vi "PR_Replace_data.vi"(7 "Boolean":bool, 8 "error in (no error)":errorcluster, 9 "Barcode_B":string, 10 "Barcode_A":string, 11 "DBlink":string="Driver={ODBC Driver 17 for SQL Server};Server=localhost\\SQLEXPRESS;Database=ZDX201;UID=labview;PWD=Dsa@54137926") -> (0 "error out":errorcluster, 1 "data":cluster{string}[](array[cluster]))   [LabVIEW 2019]
uses:
  <vilib>/addons/database/Connection.llb/DB Tools Open Connec (String).vi
  <vilib>/addons/database/Connection.llb/Conn Execute.vi
  <vilib>/addons/database/Recordset.llb/Rec Fetch Recordset Data (R).vi
  <vilib>/addons/database/Recordset.llb/Rec Destroy - Connection.vi
  <vilib>/addons/database/_DB Variant To Data/Database Variant To Data.xnode
  <vilib>/addons/database/NI_Database_API.lvlib
panel:
  out "Command 1":string="SELECT TOP (1) [id]      \n FROM [ZDX201].[dbo].[glue_data]\n where glue_workspace_id=4\nand evaluation_1 is null\norder by id desc "
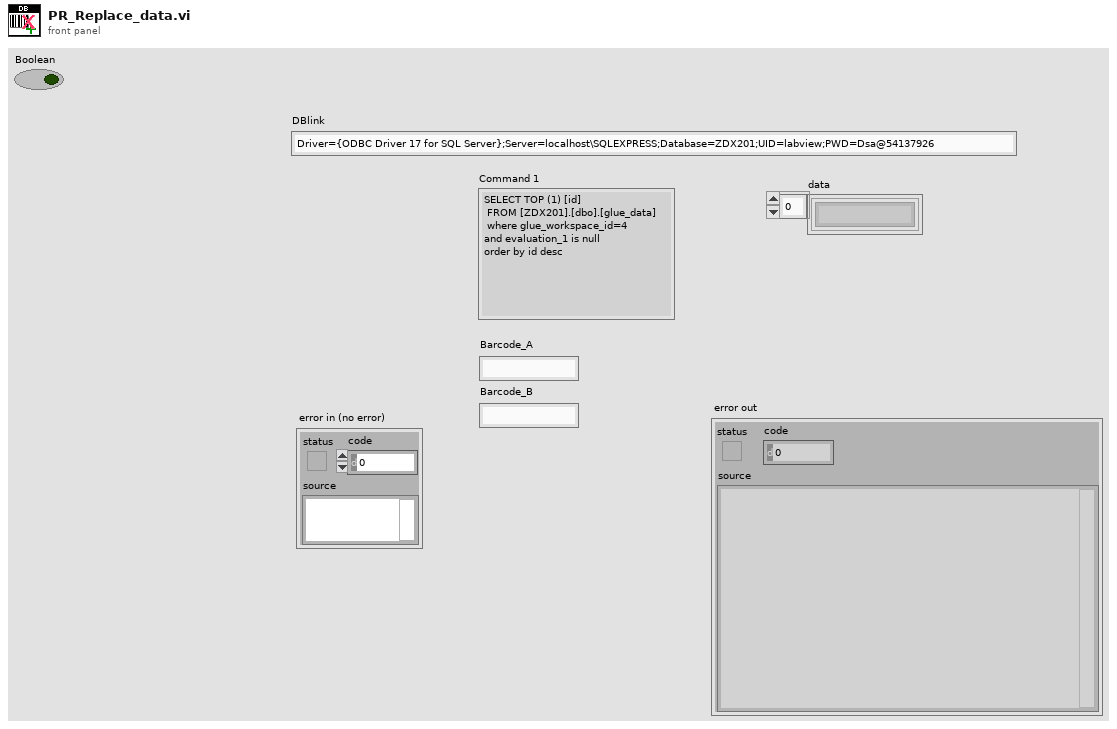
[diagram p1: front panel]
types:
  T1 = typedef "NI_Database_API.lvlib/Conn ObjectReference.ctl" = refnum<k1>
  T2 = typedef "NI_Database_API.lvlib/Rec ObjectReference.ctl" = refnum<k1>
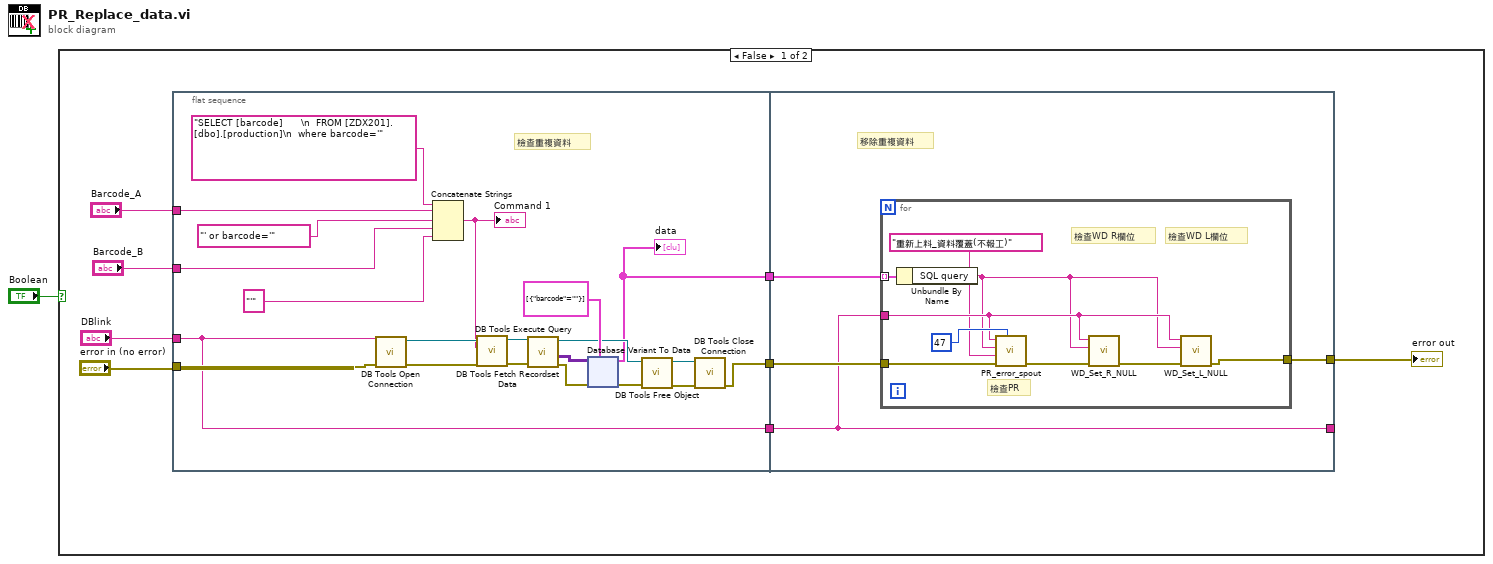
[diagram p0: block diagram]
diagram:
  n1 = case shown="False" "Boolean" {
    frame False {
      n2 = flat-sequence {
        tunnel: "DBlink" -> [w18]
        tunnel: "error in (no error)" -> [w30]
        tunnel: [w19] -> w7
        tunnel: [w18] -> w6
        tunnel: [w12] -> w5
        tunnel: "Barcode_A" -> [w11]
        tunnel: "Barcode_B" -> [w10]
        tunnel: [w74] -> _
        tunnel: w7 -> [w75]
        tunnel: w6 -> [w74]
        tunnel: w5 -> [w73]
        tunnel: [w72] -> w2
        frame #0 {
          # "檢查重複資料"
          n3 = call-poly <vilib>:"DB Tools Open Connection.vi"("error in (no error)"=w30, "connection information"=w18) -> ("error out"=w29:errorcluster, "connection reference"=w28:T1)  [unwired: 6 in]
          n4 = Concatenate Strings("SELECT [barcode]      \n  FROM [ZDX201].[dbo].[production]\n  where barcode='" ("SQL query"), w11, "' or barcode='" ("SQL query"), w10, "'" ("SQL query")) -> (w13:string)
          "Command 1" <- w13
          n5 = call-poly <vilib>:"DB Tools Execute Query.vi"("error in (no error)"=w29, "SQL query"=w13, "connection reference"=w28) -> ("error out"=w27:errorcluster, "recordset reference"=w26:T2)  [unwired: 5 in]
          n6 = call-poly <vilib>:"DB Tools Fetch Recordset Data.vi"("error in (no error)"=w27, "recordset reference"=w26) -> ("error out"=w25:errorcluster, "recordset data"=w17:variant[][], "recordset reference out"=w20:T2)  [unwired: 3 in]
          n7 = xnode "Database Variant To Data"("database variant"=w17, "error in (no error)"=w25, "type"=cluster{"barcode":string}[] [{"barcode"=""}] ("initialized array")) -> ("data"=w12:cluster{"SQL query":string}[], "error out"=w21:errorcluster)
          "data" <- w12
          n8 = call-poly <vilib>:"DB Tools Free Object.vi"("error in (no error)"=w21, "recordset reference"=w20) -> ("error out"=w22:errorcluster, "connection reference"=w23:T1)  [unwired: 8 in]
          n9 = call <vilib>:"DB Tools Close Connection.vi"("error in (no error)"=w22, "connection reference"=w23) -> ("error out"=w19:errorcluster)  [unwired: 5 in]
        }
        frame #1 {
          # "移除重複資料"
          n10 = for {
            tunnel: w75 -> [w80]
            tunnel: w74 -> [w82]
            tunnel: w73 -> [w84] mode=indexing
            tunnel: [w77] -> w72
            # "檢查PR"
            # "檢查WD L欄位"
            # "檢查WD R欄位"
            n11 = Unbundle By Name(w84) -> ("SQL query"=w81:string)
            n12 = call "PR_error_spout .vi"("[workplace_id]"=i16 47, "error in (no error)"=w80, "QC result"="重新上料_資料覆蓋(不報工)", "barcode"=w81, "DBlink"=w82) -> ("error out"=w79:errorcluster)  [unwired: 6 in]
            n13 = call "WD_Set_R_NULL.vi"("error in (no error)"=w79, "Barcode R"=w81, "DBlink"=w82) -> ("error out"=w78:errorcluster)  [unwired: 7 in, 1 out]
            n14 = call "WD_Set_L_NULL.vi"("error in (no error)"=w78, "Barcode L"=w81, "DBlink"=w82) -> ("error out"=w77:errorcluster)  [unwired: 7 in, 1 out]
          }
        }
      }
      "error out" <- w2
    }
    frame True {
    }
  }
